vi "Nelson_Find_Whale_Color.vi"(3 "error in":errorcluster, 5 "Image In":T1(plugin-control)) -> (0 "error out":errorcluster, 1 "Calibrated Centroid (Centroid 1)":cluster{"X Centroid":sgl, "Y Centroid":sgl} {"Y Centroid" format="%.2f"; "X Centroid" format="%.2f"}, 2 "Image Out":T1(plugin-control))   [LabVIEW 2014]
uses:
  <vilib>/vision/NI_Vision_Development_Module.lvlib
panel:
  out "Centroid (Centroid 1)":cluster{"X Centroid":sgl, "Y Centroid":sgl} {"Y Centroid" format="%.2f"; "X Centroid" format="%.2f"}
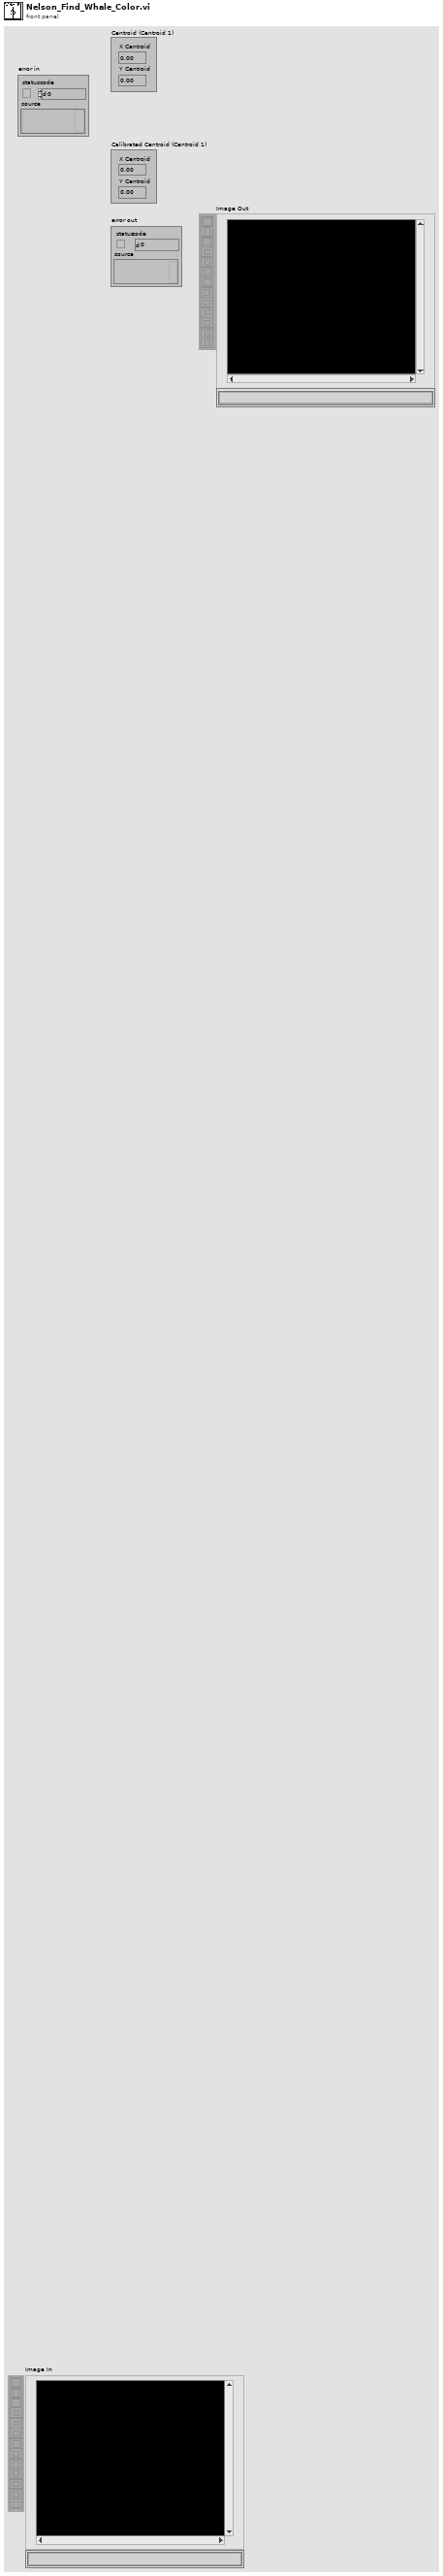
[diagram p1: front panel]
types:
  T1 = typedef "IMAQ Image.ctl" = refnum<image>
  T2 = cluster{"Global Rectangle":i32[], "Contours":cluster{"ID":enum32{"External", "Internal"}, "Type":u32, "Coordinates":i32[]}[]}
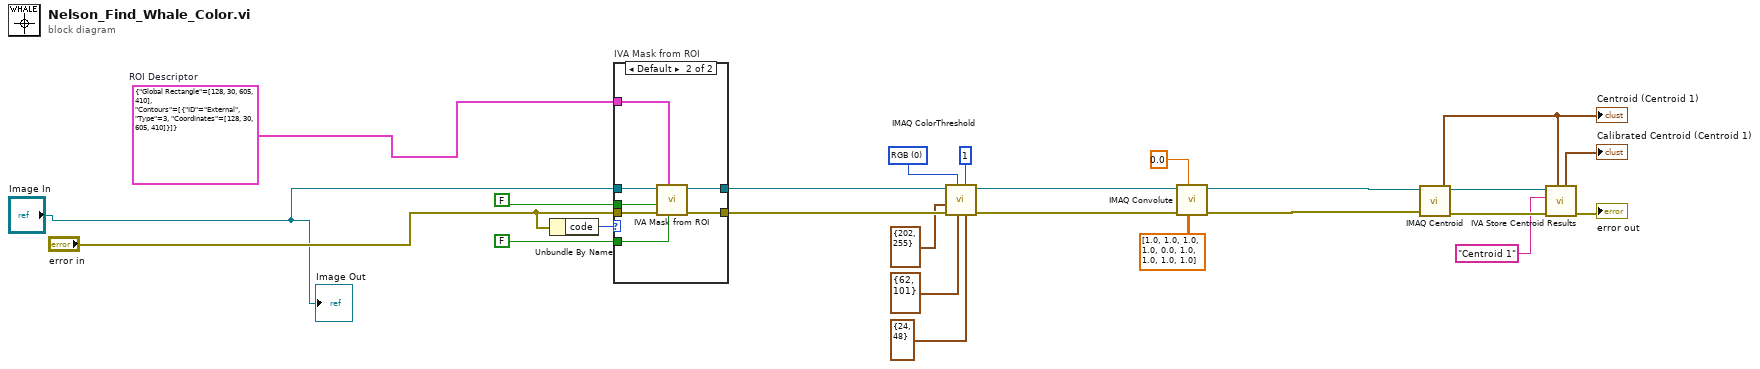
[diagram p0: block diagram]
diagram:
  w17 = u16 0 items=["RGB", "HSL", "HSV", "HSI"] ("Color Mode")
  w23 = T2 {"Global Rectangle"=[128, 30, 605, 410], "Contours"=[{"ID"=enum."External", "Type"=3, "Coordinates"=[128, 30, 605, 410]}]}  # ROI Descriptor
  n1 = Unbundle By Name("error in") -> ("code"=w19:i32)
  n2 = case "IVA Mask from ROI" shown="Default" w19 {
    tunnel: w23 -> [_ w32]
    tunnel: FALSE ("Shrink") -> [_ w31]
    tunnel: "Image In" -> [w25 w30]
    tunnel: "error in" -> [_ w29]
    tunnel: [_ w28] -> w21
    tunnel: [w25 w27] -> w13
    tunnel: FALSE ("Out / In") -> [_ w26]
    frame -1074396199, -1074396198 {
      # "Discard\nCoordinate\nSystem\nError"
    }
    frame Default {
      n3 = call <vilib>:"IVA Mask from ROI.vi"("Shrink"=w31, "ROI Descriptor"=w32, "error in (no error)"=w29, "Out / In"=w26, "Image Src"=w30) -> ("error out"=w28:errorcluster, "Image Out"=w27:T1)  [unwired: 5 out]
    }
  }
  n4 = call "IMAQ ColorThreshold"("Blue or Luma or Val or Inten Range"=cluster{"Lower value":i32, "Upper value":i32} {"Lower value"=24, "Upper value"=48}, "Replace Value"=1, "Green or Sat Range"=cluster{"Lower value":i32, "Upper value":i32} {"Lower value"=62, "Upper value"=101}, "Color Mode"=w17, "error in (no error)"=w21, "Red or Hue Range"=cluster{"Lower value":i32, "Upper value":i32} {"Lower value"=202, "Upper value"=255}, "Image Src"=w13) -> ("error out"=w12:errorcluster, "Image Dst Out"=w10:T1)  [unwired: 1 in, 2 out]
  n5 = call "IMAQ Convolute"("Kernel"=sgl[][] [[1.0, 1.0, 1.0], [1.0, 0.0, 1.0], [1.0, 1.0, 1.0]], "Divider (kernel sum)"=sgl 0.0 ("Divider"), "error in (no error)"=w12, "Image Src"=w10) -> ("error out"=w9:errorcluster, "Image Dst Out"=w5:T1)  [unwired: 3 in, 3 out]
  n6 = call "IMAQ Centroid"("error in (no error)"=w9, "Image"=w5) -> ("error out"=w7:errorcluster, "Centroid"=w3:cluster{"X Centroid":sgl, "Y Centroid":sgl})  [unwired: 1 in, 1 out]
  "Centroid (Centroid 1)" <- w3
  n7 = call <vilib>:"IVA Store Centroid Results.vi"("Centroid in"=w3, "error in (no error)"=w7, "Step Name"="Centroid 1", "Image in"=w5) -> ("error out"=→"error out":errorcluster, "Calibrated Centroid"=→"Calibrated Centroid (Centroid 1)":cluster{"X":sgl, "Y":sgl})  [unwired: 6 out]
  "Image Out" <- "Image In"
